vi "Gain_hardware.vi"(9 "error out":errorcluster, 10 "VISA resource name out":refnum<visa-resource-name>, 11 "appended array":dbl[](array[numeric])) -> (0 "Result":dbl[](array[numeric]), 2 "error out 2":errorcluster, 3 "VISA resource name out 2":refnum<visa-resource-name>)   [LabVIEW 2015]
uses:
  <vilib>/imath/engines/lvmath/Plug In/_Char/NIMS_CH_character datatype.ctl
  <vilib>/imath/engines/lvmath2/RunTimeEngine/Managers/WorkSpace/UID Generator.vi
  <vilib>/imath/engines/lvmath/Plug In/_Char/NIMS_CH_String to Character Array.vi
  <vilib>/imath/engines/lvmath2/RunTimeEngine/BuiltInFunctions/length/NIMS_length(GV).vi
  <instcachedir>/0/NIMS_length(GV)_08A3D13377FD4E4B96F5795FBF3698FA.lvgen/NIMS_length(GV)_08A3D13377FD4E4B96F5795FBF3698FA_003.vi
  <vilib>/imath/engines/lvmath2/RunTimeEngine/RunTimeType/NIMS_RunTimeType_From StrictType (excl LVString).vi
  <instcachedir>/0/NIMS_RunTimeType_From StrictType (excl LVString)_EB1C38A9BC5048DA9ABDA8F781E54D21.lvgen/NIMS_RunTimeType_From StrictType (excl LVString)_EB1C38A9BC5048DA9ABDA8F781E54D21_000.vi
  <vilib>/imath/engines/lvmath2/RunTimeEngine/LocalVariableDefStatement/MC_LocalVariableDefStatement_Display.vi
  <instcachedir>/0/NIMS_RunTimeType_From StrictType (excl LVString)_EB1C38A9BC5048DA9ABDA8F781E54D21.lvgen/NIMS_RunTimeType_From StrictType (excl LVString)_EB1C38A9BC5048DA9ABDA8F781E54D21_006.vi
  <vilib>/imath/engines/lvmath2/RunTimeEngine/RangeToken/NIMS_Range_R2 - Integer.vi
  <instcachedir>/0/NIMS_Range_R2 - Integer_396D5D4FB869421F9245109A0975AD54.lvgen/NIMS_Range_R2 - Integer_396D5D4FB869421F9245109A0975AD54_000.vi
  <vilib>/imath/engines/lvmath2/RunTimeEngine/CommandStatement/MC_CommandStatement_break.vi
  <vilib>/imath/engines/lvmath2/RunTimeEngine/IndexRead/NIMS V(S).vi
  <instcachedir>/0/NIMS V(S)_0488751826AF41519A22953C041130DC.lvgen/NIMS V(S)_0488751826AF41519A22953C041130DC_003.vi
  <vilib>/imathl/engines/lvmath/Functions/Error Handling/Create Error.vi
  <vilib>/imath/engines/lvmath/Plug In/_Char/NIMS_CH_Character 2D to String 1D.vi
  <vilib>/imath/engines/lvmath2/RunTimeEngine/BuiltInFunctions/strconcat/NIMS_strconcat.vi
  <vilib>/imath/engines/lvmath/Plug In/_Char/NIMS_CH_String CV to Character 2D.vi
  <instcachedir>/0/NIMS_CH_String CV to Character 2D_EC8CCB3F0D074D66A728E5B1D55F815A.lvgen/NIMS_CH_String CV to Character 2D_EC8CCB3F0D074D66A728E5B1D55F815A_000.vi
  <vilib>/imath/engines/lvmath2/RunTimeEngine/ErrorHandling/NIMS_Create Error From Enums.vi
  <vilib>/imath/engines/lvmath2/RunTimeEngine/RunTimeType/NIMS_RunTimeType_Get Case Value.vi
  <vilib>/imath/engines/lvmath2/RunTimeEngine/RunTimeType/NIMS_RunTimeType_To Numeric.vi
  <instcachedir>/0/NIMS_RunTimeType_To Numeric_B134FEC7BFC54ED5998F4CFD2EE98288.lvgen/NIMS_RunTimeType_To Numeric_B134FEC7BFC54ED5998F4CFD2EE98288_008.vi
  <vilib>/imath/engines/lvmath/Plug In/_Char/RunTimeType/NIMS_CH_RunTimeType_To Character 1D.vi
  <vilib>/imath/engines/lvmath/Plug In/_Char/NIMS_CH_Character 1D to U8 1D.vi
  <instcachedir>/0/NIMS_RunTimeType_From StrictType (excl LVString)_EB1C38A9BC5048DA9ABDA8F781E54D21.lvgen/NIMS_RunTimeType_From StrictType (excl LVString)_EB1C38A9BC5048DA9ABDA8F781E54D21_012.vi
  <vilib>/imath/engines/lvmath2/RunTimeSupport/NIMS_Get Row Vector_w Error - Matrix.vi
  <instcachedir>/0/NIMS_Get Row Vector_w Error - Matrix_389E9F9A4EDD452C8FD60214A0990867.lvgen/NIMS_Get Row Vector_w Error - Matrix_389E9F9A4EDD452C8FD60214A0990867_000.vi
  <vilib>/imath/engines/lvmath/Plug In/_Char/NIMS_CH_Character RV to String.vi
  <vilib>/imath/engines/lvmath2/RunTimeEngine/BuiltInFunctions/str_to_double/NIMS_str_to_double.vi
  <vilib>/imath/engines/lvmath2/RunTimeEngine/IndexReplace/NIMS V(S)=M.vi
  <instcachedir>/0/NIMS V(S)=M_9845B4AA5F6C45A990F3D6220A01B2A0.lvgen/NIMS V(S)=M_9845B4AA5F6C45A990F3D6220A01B2A0_001.vi
  <vilib>/imath/engines/lvmath2/RunTimeEngine/Managers/SymbolTable/Clear UID.vi
  <vilib>/imath/engines/lvmath2/RunTimeEngine/NodeEndStatement/NIMS_NodeEndStatement_Output.vi
  <instcachedir>/0/NIMS_NodeEndStatement_Output_53EC0D466D134D7ABD903AC30B43404B.lvgen/NIMS_NodeEndStatement_Output_53EC0D466D134D7ABD903AC30B43404B_012.vi
  <instcachedir>/0/NIMS_NodeEndStatement_Output_53EC0D466D134D7ABD903AC30B43404B.lvgen/NIMS_NodeEndStatement_Output_53EC0D466D134D7ABD903AC30B43404B_011.vi
  <instcachedir>/0/NIMS_NodeEndStatement_Output_53EC0D466D134D7ABD903AC30B43404B.lvgen/NIMS_NodeEndStatement_Output_53EC0D466D134D7ABD903AC30B43404B_000.vi
  <vilib>/imath/engines/lvmath2/RunTimeEngine/ErrorHandling/NIMS_Finalize Error.vi
  <vilib>/imath/engines/lvmath2/RunTimeEngine/Managers/SymbolTable/NIMS_WorkSpace.lvlib
panel:
  out "output":dbl[](array[numeric])
  in  "stop":bool
  out "read buffer":string
  out "Numeric":i32
  out "C":i32
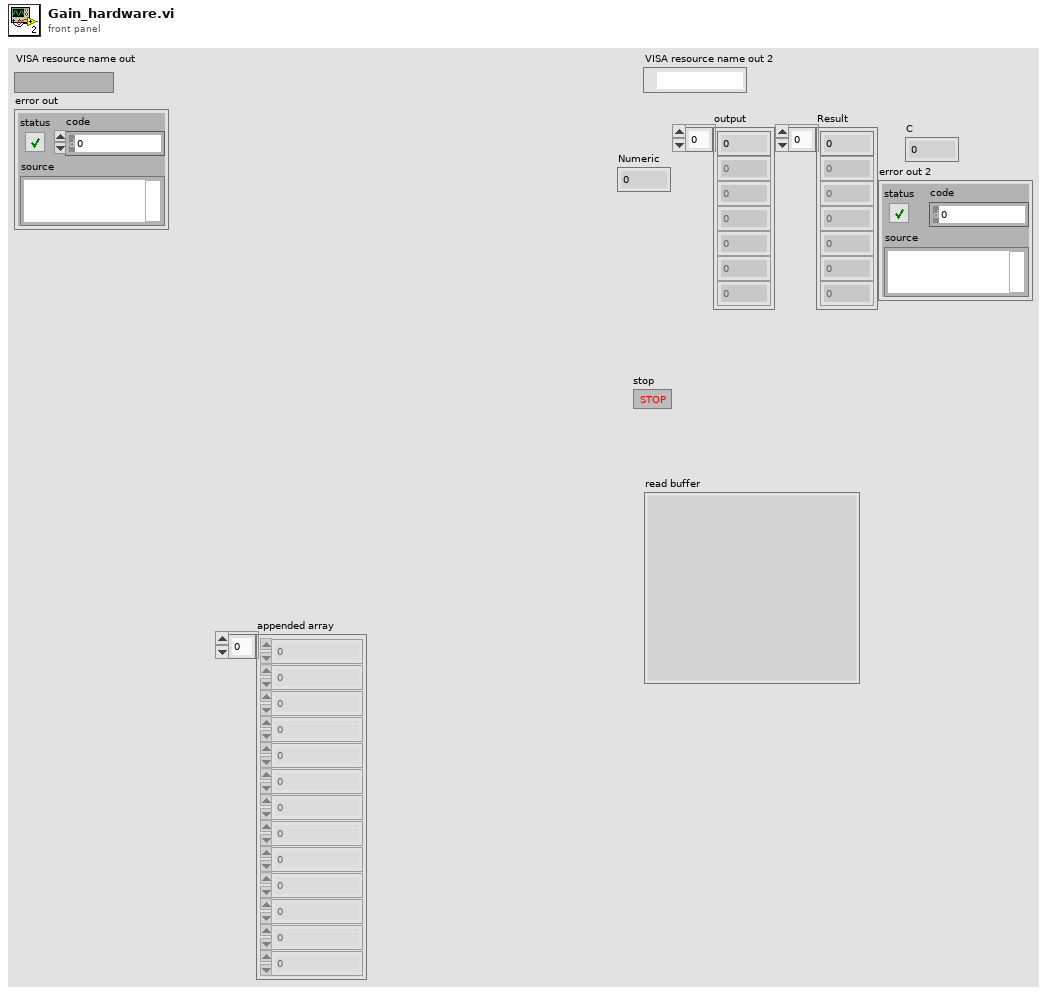
[diagram p1: front panel]
types:
  T1 = typedef "NIMS_CH_character datatype.ctl" = cluster{"Numeric":u8}
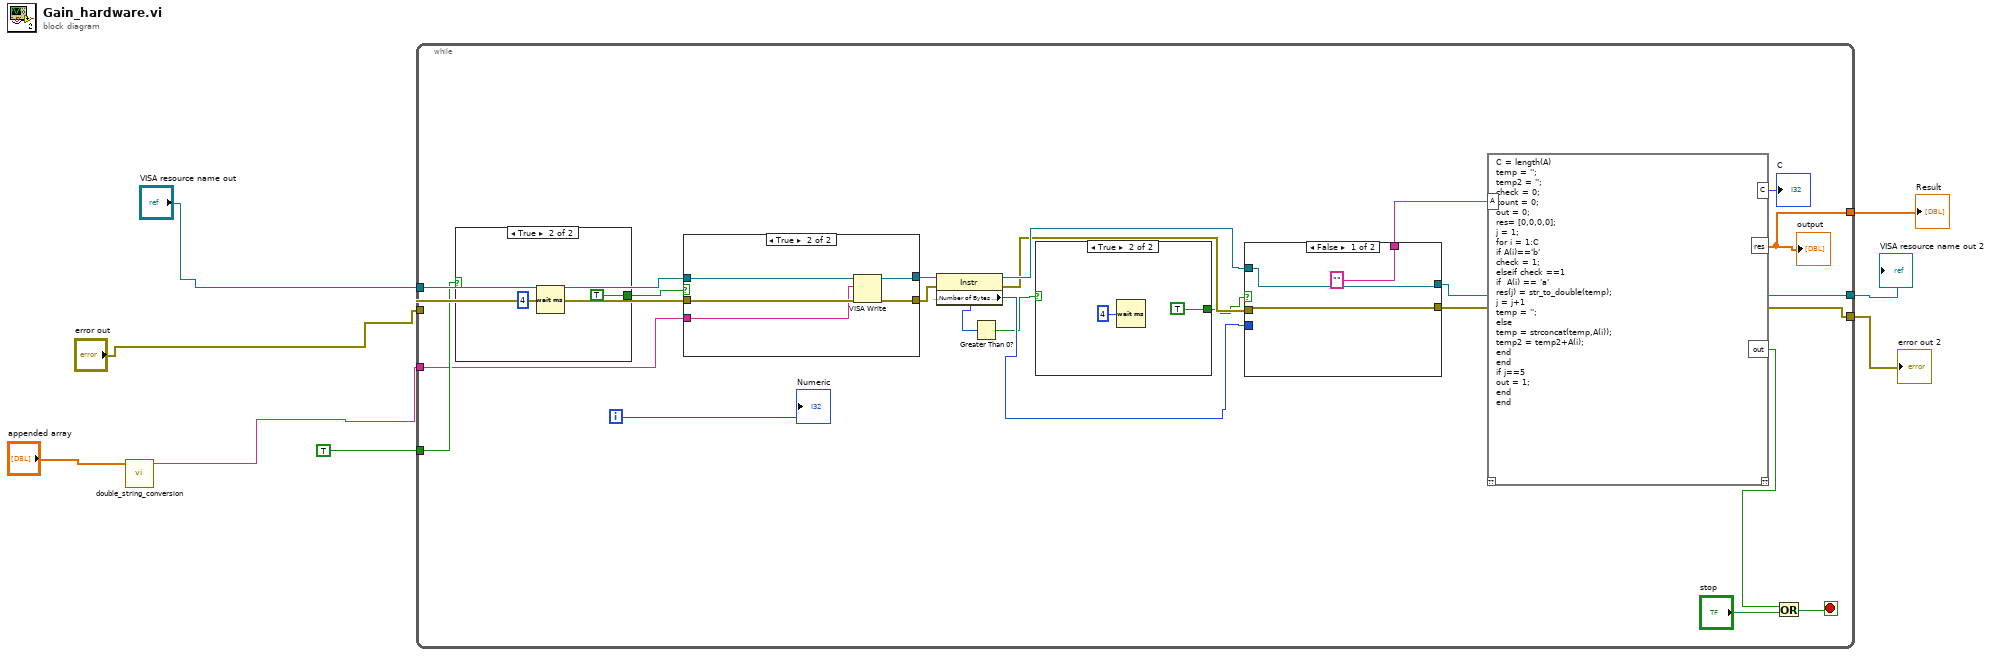
[diagram p0: block diagram]
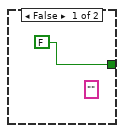
[diagram p2: hidden frame]
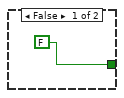
[diagram p3: hidden frame]
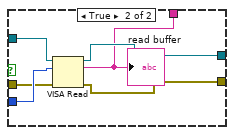
[diagram p4: hidden frame]
diagram:
  n1 = call "double_string_conversion.vi"("appended array"="appended array") -> ("concatenated string"=w4:string)  [unwired: 10 in]
  n2 = while {
    tunnel: "VISA resource name out" -> [w27]
    tunnel: "error out" -> [w26]
    tunnel: [w17] -> w8
    tunnel: [w16] -> w7
    tunnel: TRUE ("stop 2") -> [w12]
    tunnel: w4 -> [w11]
    tunnel: [w10] -> w3
    i -> [w25]
    stop <- w21 stop-if-true
    n3 = case shown="True" w12 {
      tunnel: [FALSE ("stop 2") TRUE ("stop 2")] -> w13
      frame False {
        (unwired) "" ("write buffer")
      }
      frame True {
        n4 = Wait (ms)(milliseconds to wait=u32 4) -> ()  [unwired: 1 out]
      }
    }
    n5 = case shown="True" w13 {
      tunnel: [w443 w448] -> w29
      tunnel: w27 -> [w443 w447]
      tunnel: w26 -> [w442 w446]
      tunnel: [w442 w445] -> w28
      tunnel: w11 -> [_ w444]
      frame False {
      }
      frame True {
        n6 = VISA Write(VISA resource name=w447, write buffer=w444, error in (no error)=w446) -> (VISA resource name out=w448:refnum<visa-resource-name>, error out=w445:errorcluster)  [unwired: 1 out]
      }
    }
    n7 = property class="Instr"(reference=w29, error in=w28) -> (reference out=w24:refnum<visa-resource-name>, error out=w22:errorcluster, "Serial Settings:Number of Bytes at Serial Port"=w23:u32)
    n8 = Greater Than 0?(x=w23) -> (x > 0?=w19:bool)
    n9 = case shown="True" w19 {
      tunnel: [FALSE ("stop 2") TRUE ("stop 2")] -> w18
      frame False {
      }
      frame True {
        n10 = Wait (ms)(milliseconds to wait=u32 4) -> ()  [unwired: 1 out]
      }
    }
    n11 = case shown="False" w18 {
      tunnel: [w435 w440] -> w17
      tunnel: [w434 w441] -> w16
      tunnel: w24 -> [w435 w439]
      tunnel: w23 -> [_ w438]
      tunnel: w22 -> [w434 w437]
      tunnel: ["" ("read buffer 2") w436] -> w15
      frame False {
      }
      frame True {
        n12 = VISA Read(VISA resource name=w439, byte count=w438, error in (no error)=w437) -> (VISA resource name out=w440:refnum<visa-resource-name>, read buffer=w436:string, error out=w441:errorcluster)  [unwired: 1 out]
        "read buffer" <- w436
      }
    }
    n13 = mathscript code="C = length(A)\ntemp = '';\ntemp2 = '';\ncheck = 0;\ncount = 0;\nout = 0;\nres= [0,0,0,0];\nj = 1;\nfor i = 1:C\nif A(i)=='b'\ncheck = 1;\nelseif check ==1\nif  A(i) == 'a'\nres(j) = str_to_double(temp);\nj = j+1\ntemp = '';\nelse\ntemp = strconcat(temp,A(i));\ntemp2 = temp2+A(i);\nend\nend\nif j==5\nout = 1;\nend\nend"("A"=w15) -> ("res"=w10:cdb[], "out"=w9:bool, "C"=→"C":i32)  [unwired: 1 in, 1 out]
    "output" <- w10
    n14 = Or(x=w9, y="stop") -> (x .or. y?=w21:bool)
    "Numeric" <- w25
  }
  "Result" <- w3
  "VISA resource name out 2" <- w8
  "error out 2" <- w7
